vi "Initialize VISA communication port mMc.vi"(0 "COM Port:":refnum<visa-resource-name>="COM3", 3 "error in (no error)":errorcluster, 8 "Controller address":i16=1) -> (5 "Port":T1={"P type"=1, "VISA resource name out"="", " Terminator"="\n\r", "Timeout"=300} {"Timeout" step=10; "P type" items=["none", "RS-232C", "IEEE-488.1", "IEEE-488.2"]}, 6 "Port OK":bool, 7 "Controller":string, 9 "error out":errorcluster)   [LabVIEW 2013]
uses:
  <vilib>/Instr/_visa.llb/VISA Configure Serial Port (Instr).vi
panel:
  in  "STOP":bool
  out "P wt":bool
  out "msg":string="Start this application before turning on the\ncontroller or plugging in the USB cable"
  out "232 msg":string caption="Status log"
  in  "Baud":u16(ring)=5 caption="Baud rate" items=["1200", "2400", "4800", "9600", "19200", "38400", "57600", "115200"]
  in  "cont":bool
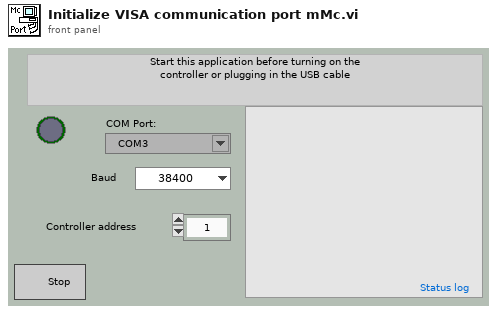
[diagram p1: front panel]
types:
  T1 = cluster{"P type":u16, "VISA resource name out":refnum<visa-resource-name>, " Terminator":string, "Timeout":i32}
  T2 = cluster{"milliseconds to wait":u32, "VISA resource name out":refnum<visa-resource-name>, string, "timeout":i32}
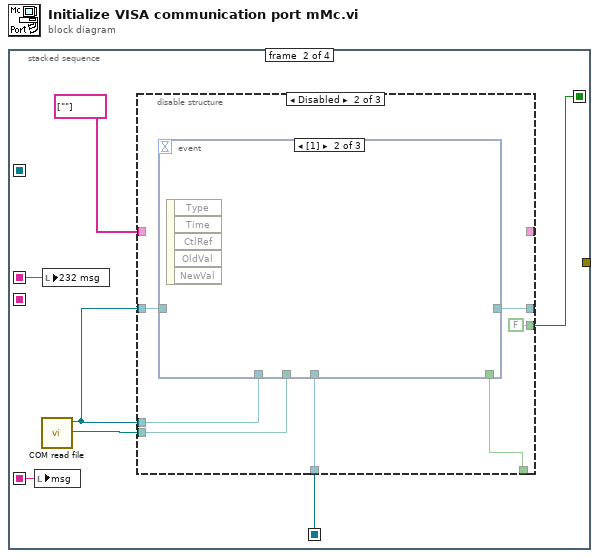
[diagram p0: block diagram]
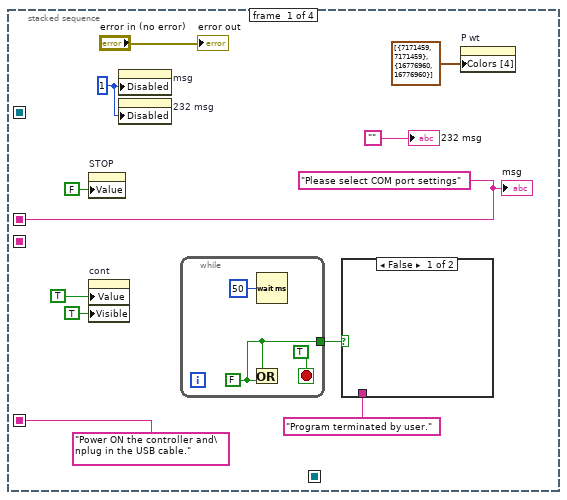
[diagram p2: hidden frame]
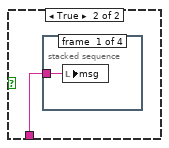
[diagram p3: hidden frame]
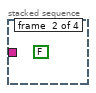
[diagram p4: hidden frame]
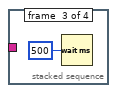
[diagram p5: hidden frame]
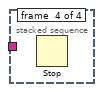
[diagram p6: hidden frame]
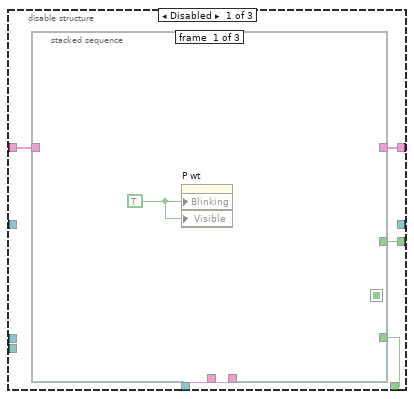
[diagram p7: hidden frame]
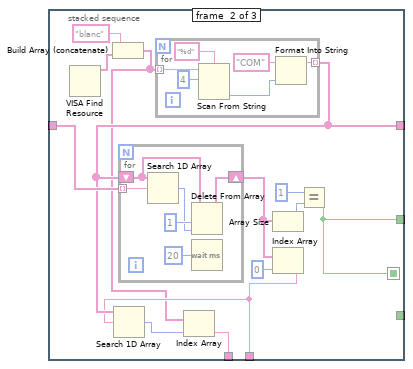
[diagram p8: hidden frame]
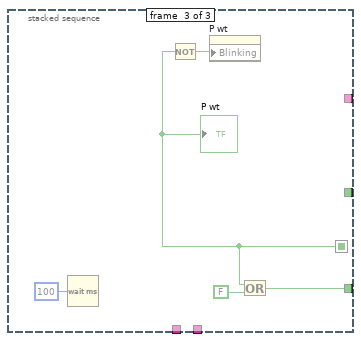
[diagram p9: hidden frame]
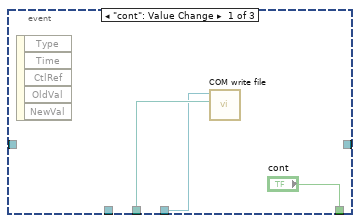
[diagram p10: hidden frame]
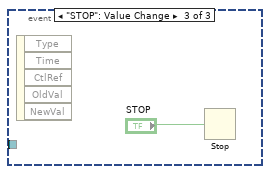
[diagram p11: hidden frame]
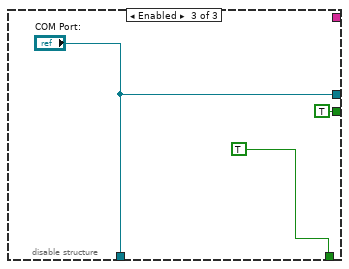
[diagram p12: hidden frame]
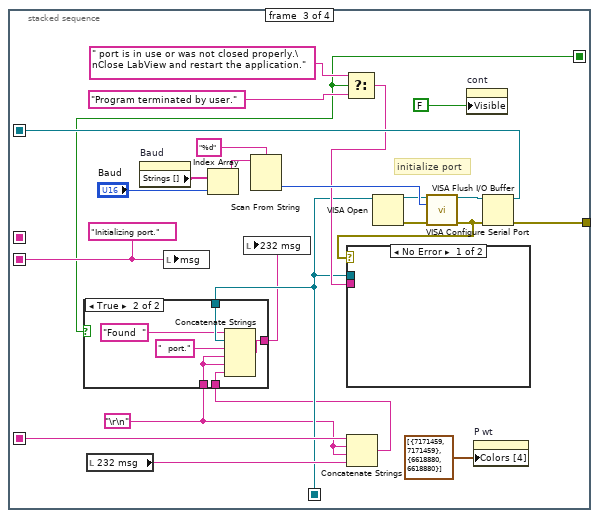
[diagram p13: hidden frame]
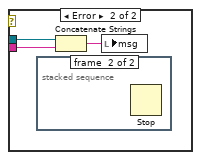
[diagram p15: hidden frame]
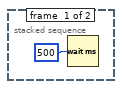
[diagram p16: hidden frame]
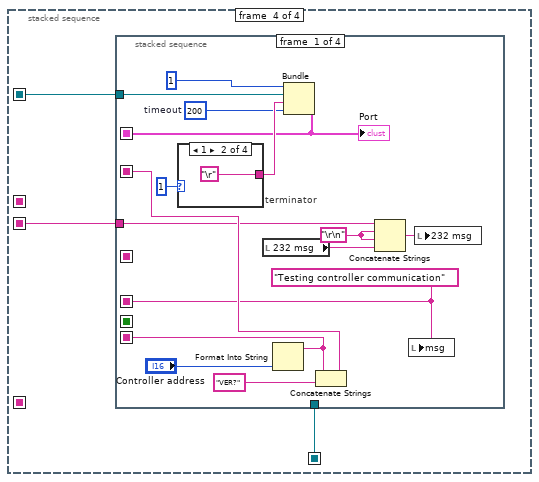
[diagram p17: hidden frame]
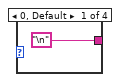
[diagram p18: hidden frame]
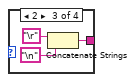
[diagram p19: hidden frame]
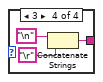
[diagram p20: hidden frame]
diagram:
  n1 = stacked-sequence {
    seq-local: [_ w23 _ _] -> [_ _ w80 w110]
    seq-local: [w8 _ _ _] -> [_ w22 _ _]
    seq-local: ["Power ON the controller and\nplug in the USB cable." ("232 msg") _ _ _] -> [_ w21 w97 _]
    seq-local: [_ _ w94 _] -> [_ _ _ w111]
    seq-local: [_ _ w86 _] -> [_ _ _ w112]
    seq-local: [_ w20 _ _] -> [_ _ w79 _]
    tunnel: [_ _ w75 _] -> _
    frame #0 {
      w8 = "Please select COM port settings" ("232 msg")
      w10 = u8 1 ("Write Attribute")
      n2 = property on="STOP" class="Bool (strict)"("Value"=FALSE ("STOP")) -> ()  [unwired: 2 in, 2 out]
      n3 = property on="cont" class="Bool (strict)"("Value"=TRUE ("cont"), "Visible"=TRUE) -> ()  [unwired: 2 in, 2 out]
      n4 = property on="msg" class="Str"("Disabled"=w10) -> ()  [unwired: 2 in, 2 out]
      n5 = property on="232 msg" class="Str"("Disabled"=w10) -> ()  [unwired: 2 in, 2 out]
      n6 = while {
        tunnel: [w15] -> w5
        stop <- TRUE stop-if-true
        w15 = FALSE ("y")
        n7 = Or(x=w15, y=w15) -> ()  [unwired: 1 out]
        n8 = Wait (ms)(milliseconds to wait=u32 50) -> ()  [unwired: 1 out]
      }
      n9 = case shown="False" w5 {
        tunnel: "Program terminated by user." -> [_ w12]
        frame False {
        }
        frame True {
          n10 = stacked-sequence {
            tunnel: w12 -> [w13 _ _ _]
            frame #0 {
              n11 = local write "msg"(w13) -> ()
            }
            frame #1 {
              (unwired) FALSE ("exit")
            }
            frame #2 {
              n12 = Wait (ms)(milliseconds to wait=u32 500) -> ()  [unwired: 1 out]
            }
            frame #3 {
              n13 = Stop() -> ()  [unwired: 1 in]
            }
          }
        }
      }
      n14 = property on="P wt" class="Bool (strict)"("Colors [4]"=cluster{u32, u32}[] [{7171459, 7171459}, {16776960, 16776960}]) -> ()  [unwired: 2 in, 2 out]
      "msg" <- w8
      "error out" <- "error in (no error)"
      "232 msg" <- ""
    }
    frame #1 {
      n15 = local write "msg"(w21) -> ()
      n16 = call "COM read file.vi"() -> ("COM file path"=w19:path, "COM port"=w18:refnum<visa-resource-name>)  [unwired: 10 in]
      n17 = local write "232 msg"(w22) -> ()
      n18 = disable-structure shown="Disabled" {
        disable-tunnel: string[] [""] -> [w29 _ _]
        disable-tunnel: [w28 _ _] -> _
        disable-tunnel: [w27 w66 "COM Port:"] -> w23
        disable-tunnel: [w26 w67 TRUE ("cont 2")] -> _
        disable-tunnel: [w25 FALSE TRUE] -> w20
        disable-tunnel: w18 -> [_ w65 _]
        disable-tunnel: [_ w64 "COM Port:"] -> _
        disable-tunnel: w18 -> [_ w63 _]
        disable-tunnel: w19 -> [_ w62 _]
        frame Disabled {
          n19 = stacked-sequence {
            seq-local: [_ w31 _] -> [_ _ w57]
            tunnel: w29 -> [_ w43 _]
            tunnel: [_ w40 _] -> w28
            tunnel: [_ w36 _] -> _
            tunnel: [_ w35 _] -> w27
            tunnel: [_ _ w58] -> w26
            tunnel: [_ w31 _] -> w25
            frame #0 {
              w30 = TRUE
              n20 = property on="P wt" class="Bool (strict)"("Blinking"=w30, "Visible"=w30) -> ()  [unwired: 2 in, 2 out]
            }
            frame #1 {
              n21 = VISA Find Resource() -> (3:w34:string[])  [unwired: 3 in, 2 out]
              n22 = Build Array (concatenate)("blanc", w34) -> (w33:string[])
              n23 = for {
                tunnel: w33 -> [w54] mode=indexing
                tunnel: [w51] -> w40 mode=indexing
                n24 = Scan From String(format string="%d", input string=w54, initial scan location=u32 4) -> (output 1=w53:i32)  [unwired: 2 in, 3 out]
                n25 = Format Into String(initial string="COM", w53) -> (resulting string=w51:string)  [unwired: 2 in, 1 out]
              }
              n26 = for {
                shift-right: [w46] -> w39
                shift-left: w40 -> [w47]
                tunnel: w43 -> [w49] mode=indexing
                n27 = Search 1D Array(1D array=w47, element=w49) -> (index of element=w45:i32)  [unwired: 1 in]
                n28 = Delete From Array(array=w47, length=1, index=w45) -> (array with subset deleted=w46:string[])  [unwired: 1 out]
                n29 = Wait (ms)(milliseconds to wait=u32 20) -> ()  [unwired: 1 out]
              }
              n30 = Array Size(array=w39) -> (size(s)=w42:i32)
              n31 = Index Array(array=w39, index=0) -> (element=w35:string)
              n32 = Search 1D Array(1D array=w40, element=w35) -> (index of element=w37:i32)  [unwired: 1 in]
              n33 = Index Array(array=w33, index=w37) -> (element=w36:string)
              n34 = Equal?(x=1, y=w42) -> (x = y?=w31:bool)
            }
            frame #2 {
              n35 = Wait (ms)(milliseconds to wait=u32 100) -> ()  [unwired: 1 out]
              n36 = Not(x=w57) -> (.not. x?=w60:bool)
              n37 = property on="P wt" class="Bool (strict)"("Blinking"=w60) -> ()  [unwired: 2 in, 2 out]
              n38 = Or(x=w57, y=FALSE) -> (x .or. y?=w58:bool)
              "P wt" <- w57
            }
          }
        }
        frame Disabled {
          n39 = event shown="[1]" {
            selector: _ -> [_ _ _]
            dyn-events: _ -> [_ _ _]
            timeout: _ -> [_ _ _]
            tunnel: ["cont" _ _] -> w67
            tunnel: [w68 _ _] -> w66
            tunnel: w65 -> [_ _ _]
            tunnel: [_ _ _] -> w64
            tunnel: w63 -> [_ _ _]
            tunnel: w62 -> [w69 _ _]
            event "cont": Value Change {
              n40 = event-data() -> ()  [unwired: 1 in, 5 out]
              n41 = call "COM write file.vi"("COM file path"=w69, "COM Port:"=w68) -> ()  [unwired: 10 in]
            }
            event #1 (no event record) {
              n42 = event-data() -> ()  [unwired: 1 in, 5 out]
            }
            event "STOP": Value Change {
              n43 = event-data() -> ()  [unwired: 1 in, 5 out]
              n44 = Stop(stop? (T)="STOP") -> ()
            }
          }
        }
        frame Enabled {
        }
      }
    }
    frame #2 {
      w94 = "Initializing port."
      w77 = "\r\n"
      # "initialize port"
      n45 = local read "232 msg"() -> (w96:string)
      n46 = property on="Baud" class="Ring (strict)"() -> ("Strings []"=w93:string[])  [unwired: 2 in, 2 out]
      n47 = local write "msg"(w94) -> ()
      n48 = Index Array(array=w93, index="Baud") -> (element=w92:string)
      n49 = Scan From String(format string="%d" ("Format String"), input string=w92) -> (output 1=w89:i32)  [unwired: 3 in, 3 out]
      n50 = Select(t=" port is in use or was not closed properly.\nClose LabView and restart the application.", s=w79, f="Program terminated by user.") -> (s? t:f=w81:string)
      n51 = Concatenate Strings(w97, w77, w77, w96) -> (w76:string)
      n52 = case shown="True" w79 {
        tunnel: w80 -> [_ w105]
        tunnel: [w99 w102] -> w78
        tunnel: w77 -> [_ w101]
        tunnel: w76 -> [w99 w100]
        frame False {
        }
        frame True {
          n53 = Concatenate Strings("Found  " ("string"), w105, "  port." ("string"), w101, w101, w100) -> (w102:string)
        }
      }
      n54 = local write "232 msg"(w78) -> ()
      n55 = VISA Open(VISA resource name=w80) -> (VISA resource name=w85:refnum<visa-resource-name>, error out=w90:errorcluster)  [unwired: 4 in]
      n56 = call-poly "VISA Configure Serial Port"("VISA resource name"=w85, "baud rate (9600)"=w89, "error in (no error)"=w90) -> ("VISA resource name out"=w88:refnum<visa-resource-name>, "error out"=w84:errorcluster)  [unwired: 11 in]
      n57 = case shown="No Error" w84 {
        tunnel: w80 -> [_ w107]
        tunnel: w81 -> [_ w106]
        frame No Error {
        }
        frame Error {
          n58 = stacked-sequence {
            frame #0 {
              n59 = Wait (ms)(milliseconds to wait=u32 500) -> ()  [unwired: 1 out]
            }
            frame #1 {
              n60 = Stop() -> ()  [unwired: 1 in]
            }
          }
          n61 = Concatenate Strings(w107, w106) -> (w108:string)
          n62 = local write "msg"(w108) -> ()
        }
      }
      n63 = property on="cont" class="Bool (strict)"("Visible"=FALSE) -> ()  [unwired: 2 in, 2 out]
      n64 = property on="P wt" class="Bool (strict)"("Colors [4]"=cluster{u32, u32}[] [{7171459, 7171459}, {6618880, 6618880}]) -> ()  [unwired: 2 in, 2 out]
      n65 = VISA Flush I/O Buffer(VISA resource name=w88, error in (no error)=w84) -> (VISA resource name out=w86:refnum<visa-resource-name>, error out=w75:errorcluster)  [unwired: 1 in]
    }
    frame #3 {
      n66 = stacked-sequence {
        seq-local: [w113 _ _ _] -> [_ w140 _ _]
        seq-local: [_ w136 _ _] -> [_ _ w161 _]
        seq-local: [_ w138 _ _] -> [_ _ w158 _]
        seq-local: [w124 _ _ _] -> [_ w139 _ _]
        seq-local: [w123 _ _ _] -> [_ _ w157 _]
        seq-local: [w114 _ _ _] -> [_ _ w153 _]
        tunnel: w112 -> [w116 _ w160 _]
        tunnel: w111 -> [w115 _ _ _]
        tunnel: w110 -> [_ _ w159 _]
        frame #0 {
          w118 = "\r\n"
          w114 = "Testing controller communication"
          w126 = 200  # timeout
          n67 = case "terminator" shown="1" u32 1 ("milliseconds to wait") {
            tunnel: ["\n" "\r" w130 w133] -> w127
            frame 0, Default {
            }
            frame 1 {
            }
            frame 2 {
              n68 = Concatenate Strings ("terminator")("\r", "\n") -> (w130:string)
            }
            frame 3 {
              n69 = Concatenate Strings ("terminator")("\n", "\r") -> (w133:string)
            }
          }
          n70 = local read "232 msg"() -> (w117:string)
          n71 = Format Into String("Controller address") -> (resulting string=w123:string)  [unwired: 3 in, 1 out]
          n72 = Bundle("milliseconds to wait"=u32 1, "VISA resource name out"=w116, w127, "timeout"=w126) -> (w113:T2)  [unwired: 1 in]
          "Port" <- w113
          n73 = Concatenate Strings ("terminator")(w123, "VER?" ("Command")) -> (w124:string)
          n74 = Concatenate Strings(w115, w118, w118, w117) -> (w119:string)
          n75 = local write "msg"(w114) -> ()
          n76 = local write "232 msg"(w119) -> ()
        }
        frame #1 {
          # "read controller version"
          n77 = Tick Count (ms)() -> (millisecond timer value=w137:u32)
          n78 = while {
            tunnel: w140 -> [w152]
            tunnel: w139 -> [w148]
            tunnel: [w151] -> w138
            tunnel: [w141] -> w136
            tunnel: w137 -> [w147]
            stop <- w143 stop-if-true
            n79 = call "DelayPiezo.vi"("old timer value"=w147, "milliseconds to wait"=200) -> ("elapsed time"=w145:u32, "error out"=w149:errorcluster)  [unwired: 5 in, 1 out]
            n80 = Greater?(x=w145, y=3000) -> (0:w142:bool)
            n81 = call "Communication VISA mMc.vi"("Port"=w152, "Command"=w148, "error in (no error)"=w149) -> ("Return"=w151:string)  [unwired: 3 in, 3 out]
            n82 = String Length(string=w151) -> (length=w150:i32)
            n83 = Greater Than 0?(x=w150) -> (x > 0?=w141:bool)
            n84 = Or(x=w141, y=w142) -> (x .or. y?=w143:bool)
          }
          "Port OK" <- w136
        }
        frame #2 {
          w155 = "\r\n"
          n85 = local read "232 msg"() -> (w154:string)
          n86 = case shown="True" w161 {
            tunnel: w160 -> [w162 _]
            tunnel: w159 -> [_ w165]
            tunnel: w158 -> [_ w167]
            tunnel: w157 -> [_ w164]
            frame False {
              n87 = VISA Close(VISA resource name=w162) -> ()  [unwired: 1 in, 1 out]
              n88 = local write "msg"("Controller did not respond to a VER? command.\nMake sure the addrss and the Baud rate are correct." ("msg")) -> ()
            }
            frame True {
              n89 = Concatenate Strings("Found controller # " ("msg"), w164, " on port " ("msg"), w165, "\r\n", w167) -> (w169:string)
              n90 = local write "msg"(w169) -> ()
              "Controller" <- w165
            }
          }
          n91 = Concatenate Strings(w153, w155, w155, w154) -> (w156:string)
          n92 = local write "232 msg"(w156) -> ()
        }
        frame #3 {
          n93 = Wait (ms)(milliseconds to wait=u32 1000) -> ()  [unwired: 1 out]
        }
      }
    }
  }
